vi "Autosampler Status Update.vi"(8 "error in (no error)":errorcluster, 10 "Autosampler Status":T1, 11 "Application in":refnum<class "Application.lvclass">) -> (0 "error out":errorcluster, 3 "Application out":refnum<class "Application.lvclass">)   [LabVIEW 2023, in "Application.lvlib" / "Application.lvclass"]
uses:
  Application.lvclass
  Hardware/Autosampler/Autosampler Status.ctl
  Hardware/Autosampler/Autosampler State2.ctl
  Application.lvclass/Application.ctl
  User Interface/Main Window Messages/Autosampler Status Update Msg/Autosampler Status Update Msg.lvclass/Autosampler Status Update Msg.ctl
  <vilib>/ActorFramework/Message Enqueuer/Message Enqueuer.lvclass/Message Enqueuer.ctl
  <vilib>/ActorFramework/Message Enqueuer/Enqueue.vi
  User Interface/Main Window Messages/Autosampler Status Update Msg/Autosampler Status Update Msg.lvclass
  <vilib>/ActorFramework/Message Priority Queue/Priority Enqueue.vi
  <vilib>/ActorFramework/Message Enqueuer/Message Enqueuer.lvclass
  Hardware/Autosampler/Autosampler.lvlib
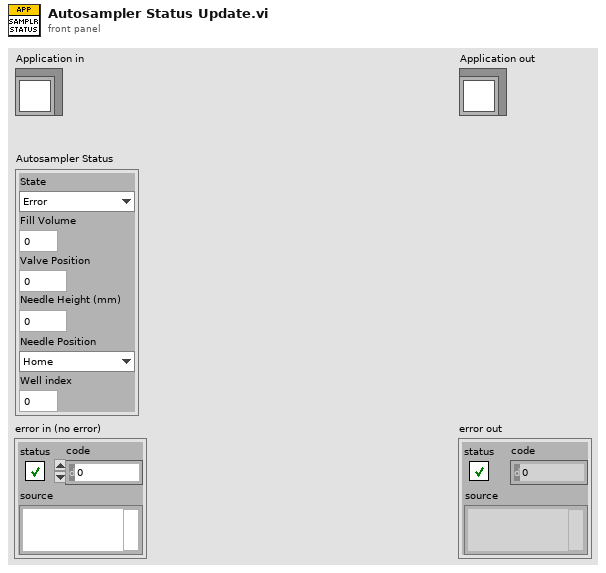
[diagram p1: front panel]
types:
  T1 = typedef "Autosampler.lvlib/Autosampler Status.ctl" = cluster{"State":T2, "Fill Volume":u16, "Valve Position":u16, "Needle Height (mm)":u16, "Needle Position":enum16{"Home", "Well", "Wash Port"}, "Well index":u16}
  T2 = typedef "Autosampler.lvlib/Autosampler State2.ctl" = enum16{"Error", "Idle", "Positioning", "Pumping", "Shaking", "Washing", "Priming"}
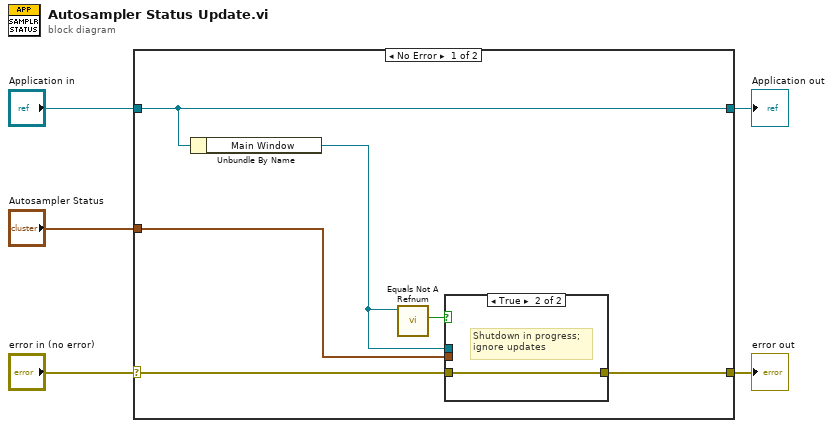
[diagram p0: block diagram]
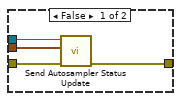
[diagram p2: hidden frame]
diagram:
  n1 = case shown="No Error" "error in (no error)" {
    selector: "error in (no error)" -> [w9 w18]
    tunnel: [w8 w18] -> w4
    tunnel: [w11 w17] -> w2
    tunnel: "Application in" -> [w11 w17]
    tunnel: "Autosampler Status" -> [w10 _]
    frame No Error {
      n2 = Unbundle By Name(w11) -> ("Main Window"=w7:refnum<class "Message Enqueuer.lvclass">)
      n3 = call <vilib>:"Equals Not A Refnum.vi"("Message Enqueuer"=w7) -> ("Not a refnum?"=w6:bool)  [unwired: 10 in]
      n4 = case shown="True" w6 {
        tunnel: w10 -> [w15 _]
        tunnel: w9 -> [w14 w16]
        tunnel: [w13 w16] -> w8
        tunnel: w7 -> [w12 _]
        frame False {
          n5 = call "Send Autosampler Status Update.vi"("error in (no error)"=w14, "Autosampler Status"=w15, "Message Enqueuer"=w12) -> ("error out"=w13:errorcluster)  [unwired: 7 in, 1 out]
        }
        frame True {
          # "Shutdown in progress;\nignore updates"
        }
      }
    }
    frame Error {
    }
  }
  "error out" <- w4
  "Application out" <- w2
